vi "Injection_time_Decrypt_Labview.vi"() -> ()   [LabVIEW 2022 SP3]
panel:
  out "Injection Second":i32
  out "Injection Minute":i32
  out "Injection Hour":i32
  in  "Encrypt Injection Time":string
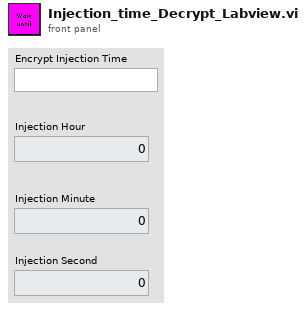
[diagram p1: front panel]
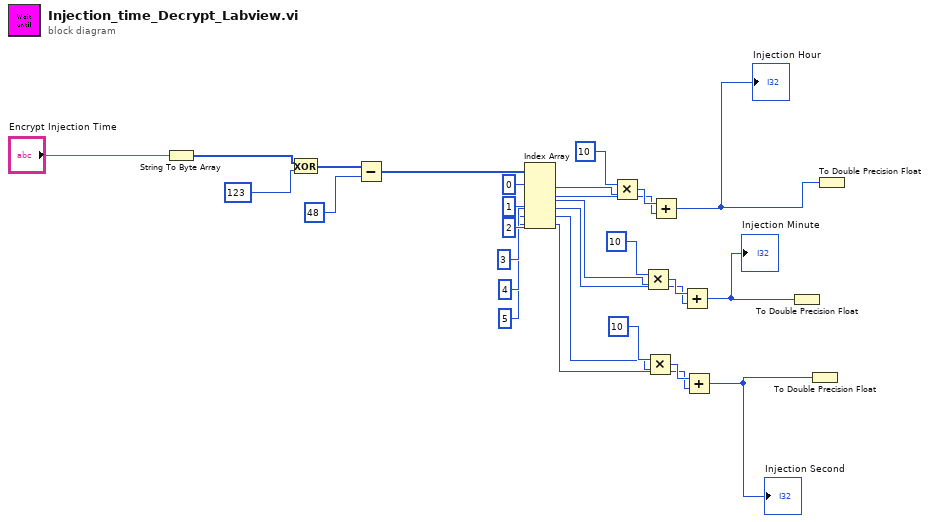
[diagram p0: block diagram]
diagram:
  n1 = String To Byte Array(string="Encrypt Injection Time") -> (unsigned byte array=w27:u8[])
  n2 = Exclusive Or(1:123, 2:w27) -> (0:w16:i32[])
  n3 = Subtract(x=w16, y=48) -> (x-y=w14:i32[])
  n4 = Index Array(array=w14, index #1=0 ("索引"), index #2=1 ("索引"), index #3=2 ("索引"), index #4=3 ("索引"), index #5=4 ("索引"), index #6=5 ("索引")) -> (element #1=w12:i32, element #2=w17:i32, element #3=w9:i32, element #4=w8:i32, element #5=w5:i32, element #6=w4:i32)
  n5 = Multiply(x=10 ("y"), y=w12) -> (x*y=w18:i32)
  n6 = Multiply(x=10 ("y"), y=w9) -> (x*y=w11:i32)
  n7 = Multiply(x=10 ("y"), y=w5) -> (x*y=w7:i32)
  n8 = Add(x=w18, y=w17) -> (x+y=w3:i32)
  "Injection Hour" <- w3
  n9 = Add(x=w11, y=w8) -> (x+y=w2:i32)
  "Injection Minute" <- w2
  n10 = Add(x=w7, y=w4) -> (x+y=w1:i32)
  "Injection Second" <- w1
  n11 = To Double Precision Float(number=w2) -> ()  [unwired: 1 out]
  n12 = To Double Precision Float(number=w1) -> ()  [unwired: 1 out]
  n13 = To Double Precision Float(number=w3) -> ()  [unwired: 1 out]
